vi "Depth2ColorImage.vi"(11 "Depth":u16[][](array[numeric])) -> (3 "HSV Image":picture)   [LabVIEW 2015]
uses:
  <vilib>/picture/picture.llb/Draw True-Color Pixmap.vi
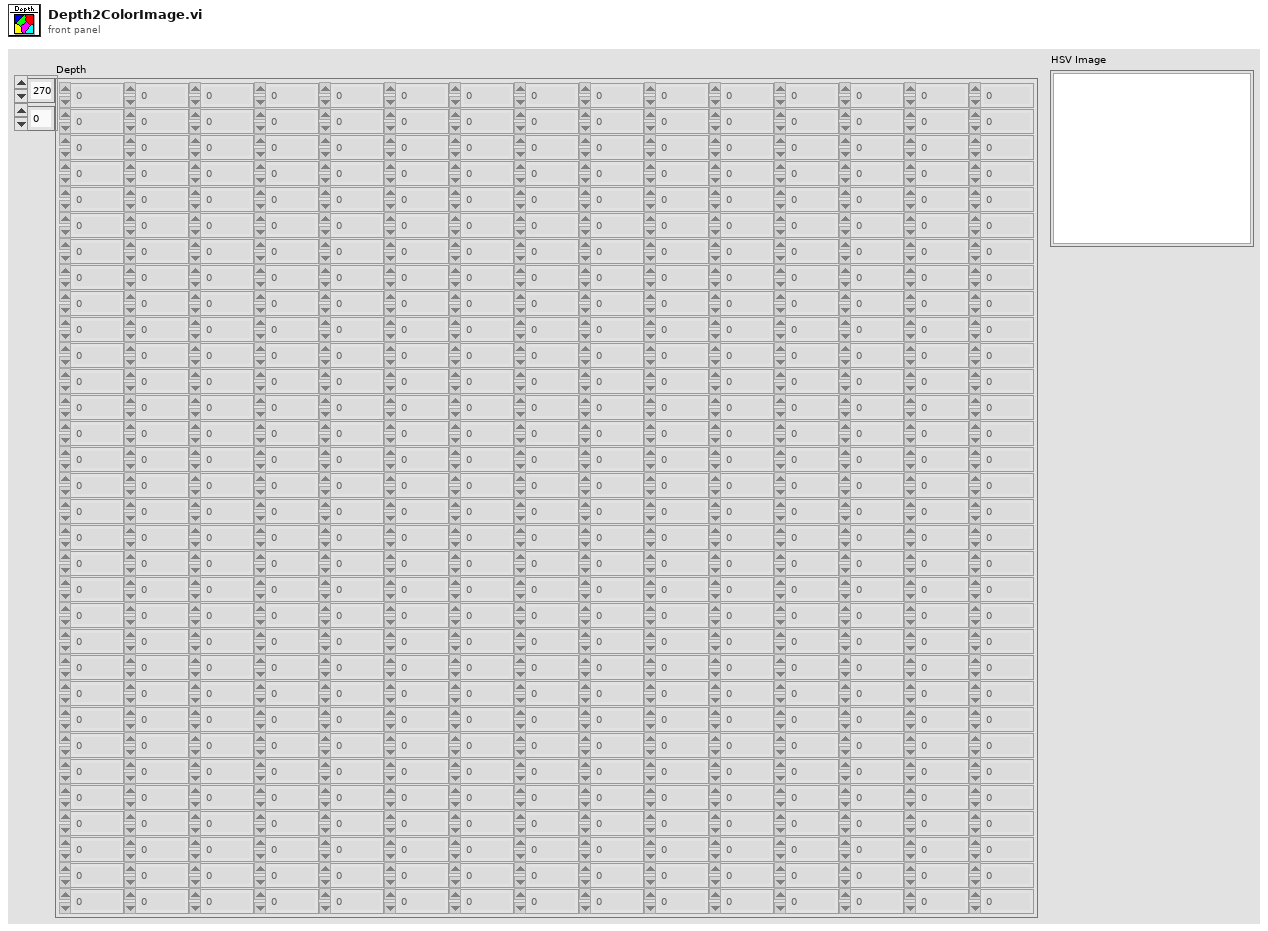
[diagram p1: front panel]
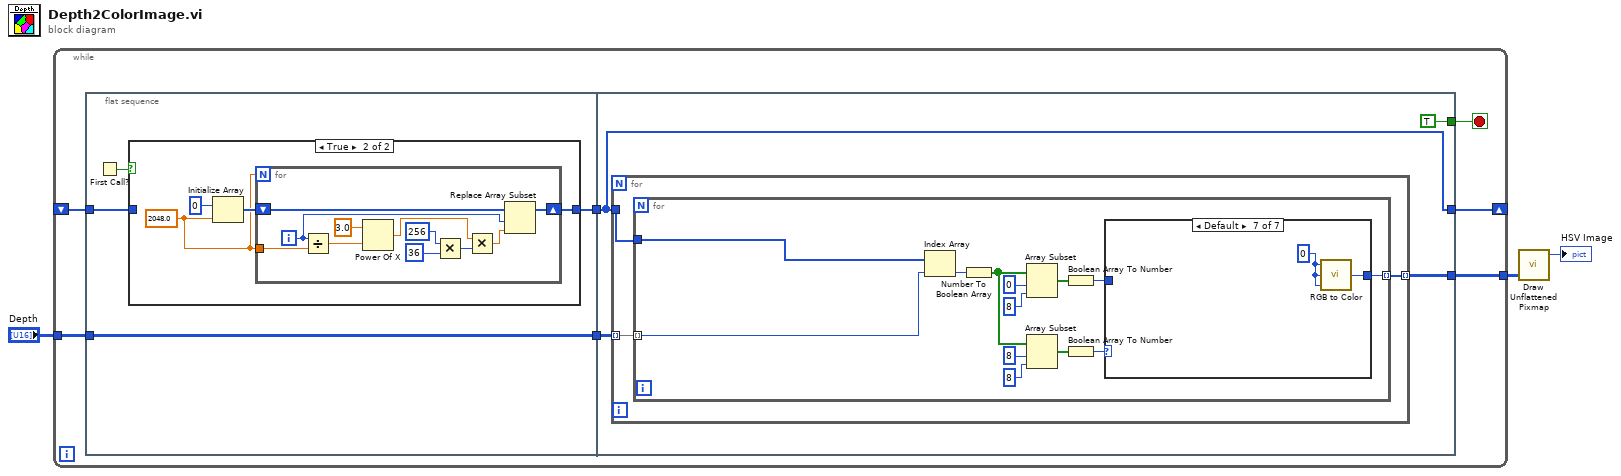
[diagram p0: block diagram]
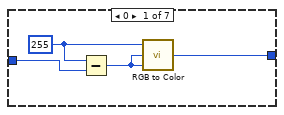
[diagram p3: hidden frame]
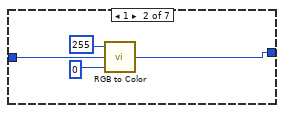
[diagram p4: hidden frame]
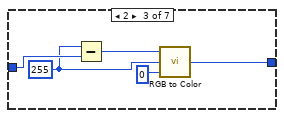
[diagram p5: hidden frame]
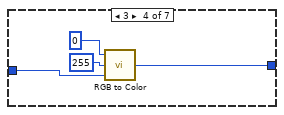
[diagram p6: hidden frame]
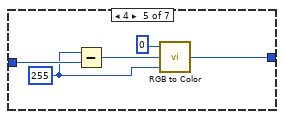
[diagram p7: hidden frame]
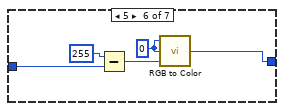
[diagram p8: hidden frame]
diagram:
  n1 = while {
    shift-right: [w9] -> _
    shift-left: _ -> [w8]
    tunnel: "Depth" -> [w6]
    tunnel: [w4] -> w2
    stop <- w5 stop-if-true
    n2 = flat-sequence {
      tunnel: [w13] -> w10
      tunnel: w8 -> [w12]
      tunnel: [w11] -> w7
      tunnel: w6 -> [w11]
      tunnel: w10 -> [w33]
      tunnel: [w33] -> w9
      tunnel: w7 -> [w34]
      tunnel: [TRUE] -> w5
      tunnel: [w31] -> w4
      frame #0 {
        n3 = First Call?() -> (First Call?: T/F=w14:bool)
        n4 = case shown="True" w14 {
          tunnel: [w15 w16] -> w13
          tunnel: w12 -> [w15 _]
          frame False {
          }
          frame True {
            w17 = 2048.0
            n5 = Initialize Array(u16 0 ("element"), w17) -> (w18:u16[])
            n6 = for {
              N: w17 -> [_]
              shift-right: [w21] -> w16
              shift-left: w18 -> [w30]
              tunnel: w17 -> [w28]
              i -> [w29]
              n7 = Divide(x=w29, y=w28) -> (x/y=w27:dbl)
              n8 = Power Of X(1:w27, 2:3.0 ("y")) -> (0:w25:dbl)
              n9 = Multiply(x=256, y=36) -> (x*y=w22:i32)
              n10 = Multiply(x=w25, y=w22) -> (x*y=w20:dbl)
              n11 = Replace Array Subset(array=w30, new element=w20, index=w29) -> (w21:u16[])
            }
          }
        }
      }
      frame #1 {
        n12 = for {
          tunnel: w34 -> [w37] mode=indexing
          tunnel: w33 -> [w36]
          tunnel: [w35] -> w31 mode=indexing
          n13 = for {
            tunnel: w37 -> [w38] mode=indexing
            tunnel: w36 -> [w50]
            tunnel: [w40] -> w35 mode=indexing
            n14 = Index Array(array=w50, index=w38) -> (element=w39:u16)
            n15 = Number To Boolean Array(number=w39) -> (Boolean array=w47:bool[])
            n16 = Array Subset(array=w47, index=0, length=8) -> (w44:bool[])
            n17 = Array Subset(array=w47, index=8, length=8) -> (w43:bool[])
            n18 = Boolean Array To Number(Boolean array=w44) -> (number=w41:u32)
            n19 = Boolean Array To Number(Boolean array=w43) -> (number=w42:u32)
            n20 = case shown="Default" w42 {
              tunnel: w41 -> [w53 w56 w63 w64 w70 w76 _]
              tunnel: [w51 w57 w62 w67 w72 w77 w79] -> w40
              frame 0 {
                w54 = 255
                n21 = Subtract(x=w54, y=w53) -> (x-y=w52:u32)
                n22 = call <vilib>:"RGB to Color.vi"("B"=w52, "G"=w52, "R"=w54) -> ("Color"=w51:u32)
              }
              frame 1 {
                n23 = call <vilib>:"RGB to Color.vi"("B"=0, "G"=w56, "R"=255) -> ("Color"=w57:u32)
              }
              frame 2 {
                w60 = 255
                n24 = Subtract(x=w60, y=w63) -> (x-y=w61:u32)
                n25 = call <vilib>:"RGB to Color.vi"("B"=0, "G"=w60, "R"=w61) -> ("Color"=w62:u32)
              }
              frame 3 {
                n26 = call <vilib>:"RGB to Color.vi"("B"=w64, "G"=255, "R"=0) -> ("Color"=w67:u32)
              }
              frame 4 {
                w68 = 255
                n27 = Subtract(x=w68, y=w70) -> (x-y=w69:u32)
                n28 = call <vilib>:"RGB to Color.vi"("B"=w68, "G"=w69, "R"=0) -> ("Color"=w72:u32)
              }
              frame 5 {
                w74 = 0
                n29 = Subtract(x=255, y=w76) -> (x-y=w73:u32)
                n30 = call <vilib>:"RGB to Color.vi"("B"=w73, "G"=w74, "R"=w74) -> ("Color"=w77:u32)
              }
              frame Default {
                w78 = 0
                n31 = call <vilib>:"RGB to Color.vi"("B"=w78, "G"=w78, "R"=w78) -> ("Color"=w79:u32)
              }
            }
          }
        }
      }
    }
  }
  n32 = call-poly <vilib>:"Draw Unflattened Pixmap.vi"("data (RGB format)"=w2) -> ("new picture"=→"HSV Image":picture)  [unwired: 8 in]
